vi "RunFullWormContinuousGWN.vi"() -> ()   [LabVIEW 2019]
uses:
  Parameters.ctl
  FullWormGWNClass/FullWormGWNInputCluster.ctl
  FullWormGWN.lvclass
  C:/Users/mochil/Dropbox/LeiferShaevitz/Github/ProjectAPI/LabviewVIs/StimulusObject.lvclass
panel:
  in  "FullWormGWNInputCluster":T1={"offset (red uW/mm^2m, blue is negative)"=0.0, "correlation time (s)"=0.5, "standard deviation (red uW/mm^2)"=70.0, "Max blue stimulus (uW/mm^2)"=130.0, "Max red stimulus (uW/mm^2)"=45.0, "dot radius (mm)"=0.3} {"Max red stimulus (uW/mm^2)" format="%#_13g"; "Max blue stimulus (uW/mm^2)" format="%#_13g"; "standard deviation (red uW/mm^2)" format="%#_13g"; "correlation time (s)" format="%#_13g"; "offset (red uW/mm^2m, blue is negative)" format="%#_13g"}
  out "error IO":errorcluster
  in  "Start":bool
  in  "Wait Before Recording (s)":u32
  in  "SSH password":string
  in  "SSH user name":string
  in  "Last Experiment of the Day":bool
  in  "Tags":string
  out "Parameters":T2 {"FW_WormLengthSD" format="%#.6e"}
  # "Faux Worm Drawing"
  # "Tracking"
  # "Temporal Calibration"
  # "Stimulus Generation"
  # "Median Filtering"
  # "Experimental Settings"
  # "Camera and Projector Settings"
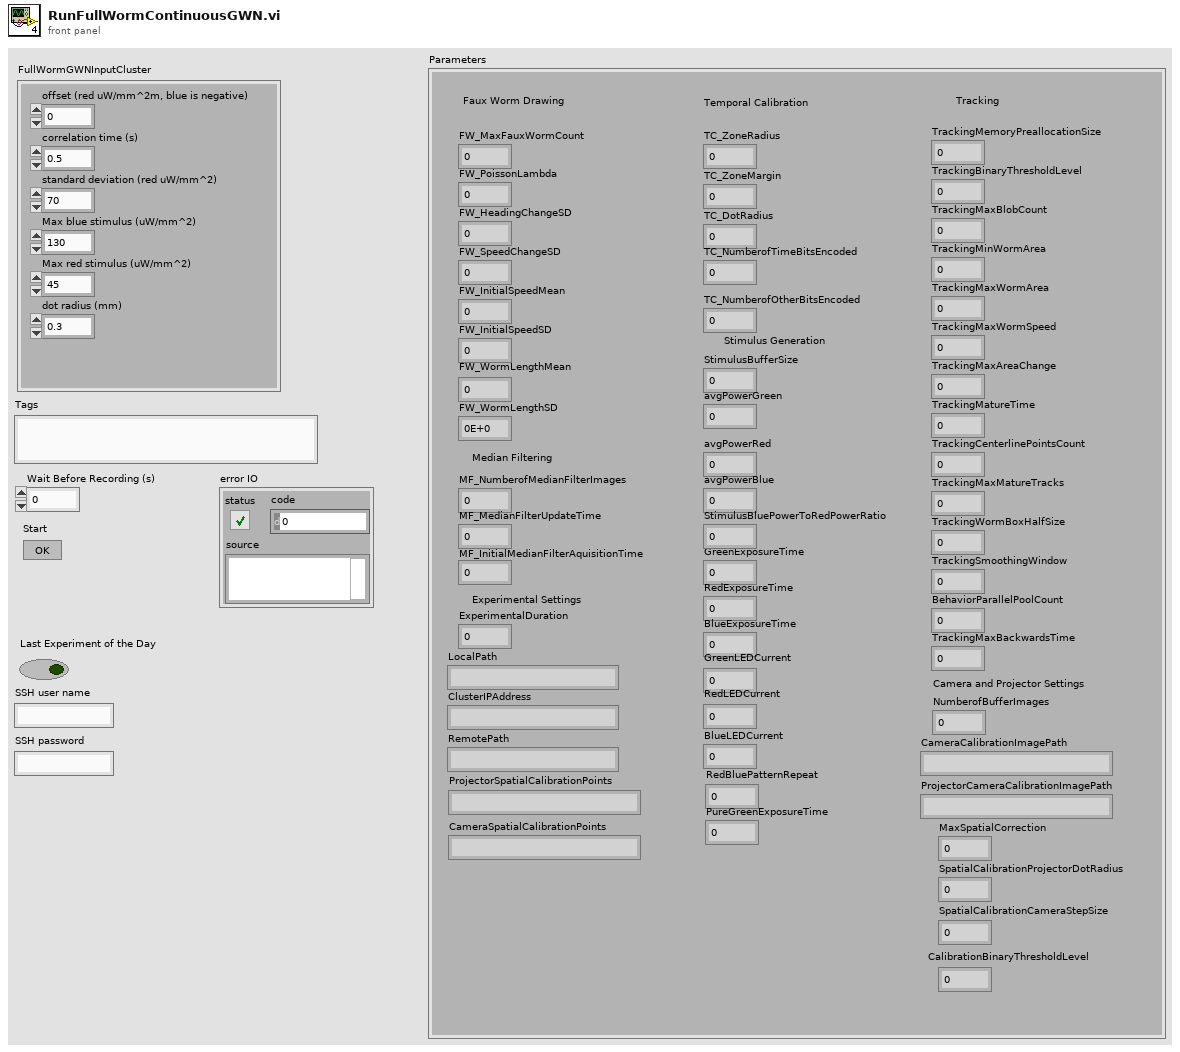
[diagram p1: front panel]
types:
  T1 = typedef "FullWormGWN.lvclass/FullWormGWNInputCluster.ctl" = cluster{"offset (red uW/mm^2m, blue is negative)":sgl, "correlation time (s)":sgl, "standard deviation (red uW/mm^2)":sgl, "Max blue stimulus (uW/mm^2)":sgl, "Max red stimulus (uW/mm^2)":sgl, "dot radius (mm)":sgl}
  T2 = typedef "Parameters.ctl" = cluster{"FW_MaxFauxWormCount":i32, "FW_PoissonLambda":dbl, "FW_HeadingChangeSD":dbl, "FW_SpeedChangeSD":dbl, "FW_InitialSpeedMean":dbl, "FW_InitialSpeedSD":dbl, "FW_WormLengthMean":dbl, "FW_WormLengthSD":dbl, "MF_NumberofMedianFilterImages":i32, "MF_MedianFilterUpdateTime":i32, "MF_InitialMedianFilterAquisitionTime":dbl, "ExperimentalDuration":i32, "TC_ZoneRadius":i32, "TC_ZoneMargin":i32, "TC_DotRadius":dbl, "TC_NumberofTimeBitsEncoded":i32, "TC_NumberofOtherBitsEncoded":i32, "NumberofBufferImages":sgl, "CameraCalibrationImagePath":string, "ProjectorCameraCalibrationImagePath":string, "StimulusBufferSize":i32, "TrackingMemoryPreallocationSize":i32, "TrackingBinaryThresholdLevel":sgl, "TrackingMaxBlobCount":i32, "TrackingMinWormArea":dbl, "TrackingMaxWormArea":dbl, "TrackingMaxWormSpeed":dbl, "TrackingMaxAreaChange":dbl, "TrackingMatureTime":i32, "TrackingCenterlinePointsCount":i32, "TrackingMaxMatureTracks":i32, "TrackingWormBoxHalfSize":i32, "TrackingSmoothingWindow":i32, "BehaviorParallelPoolCount":i32, "LocalPath":string, "GreenExposureTime":i32, "RedExposureTime":i32, "BlueExposureTime":i32, "ClusterIPAddress":string, "RemotePath":string, "GreenLEDCurrent":u8, "RedLEDCurrent":u8, "BlueLEDCurrent":u8, "avgPowerGreen":sgl, "avgPowerRed":sgl, "avgPowerBlue":sgl, "StimulusBluePowerToRedPowerRatio":sgl, "TrackingMaxBackwardsTime":i32, "MaxSpatialCorrection":dbl, "ProjectorSpatialCalibrationPoints":string, "SpatialCalibrationProjectorDotRadius":i32, "SpatialCalibrationCameraStepSize":dbl, "CameraSpatialCalibrationPoints":string, "CalibrationBinaryThresholdLevel":dbl, "RedBluePatternRepeat":i32, "PureGreenExposureTime":i32}
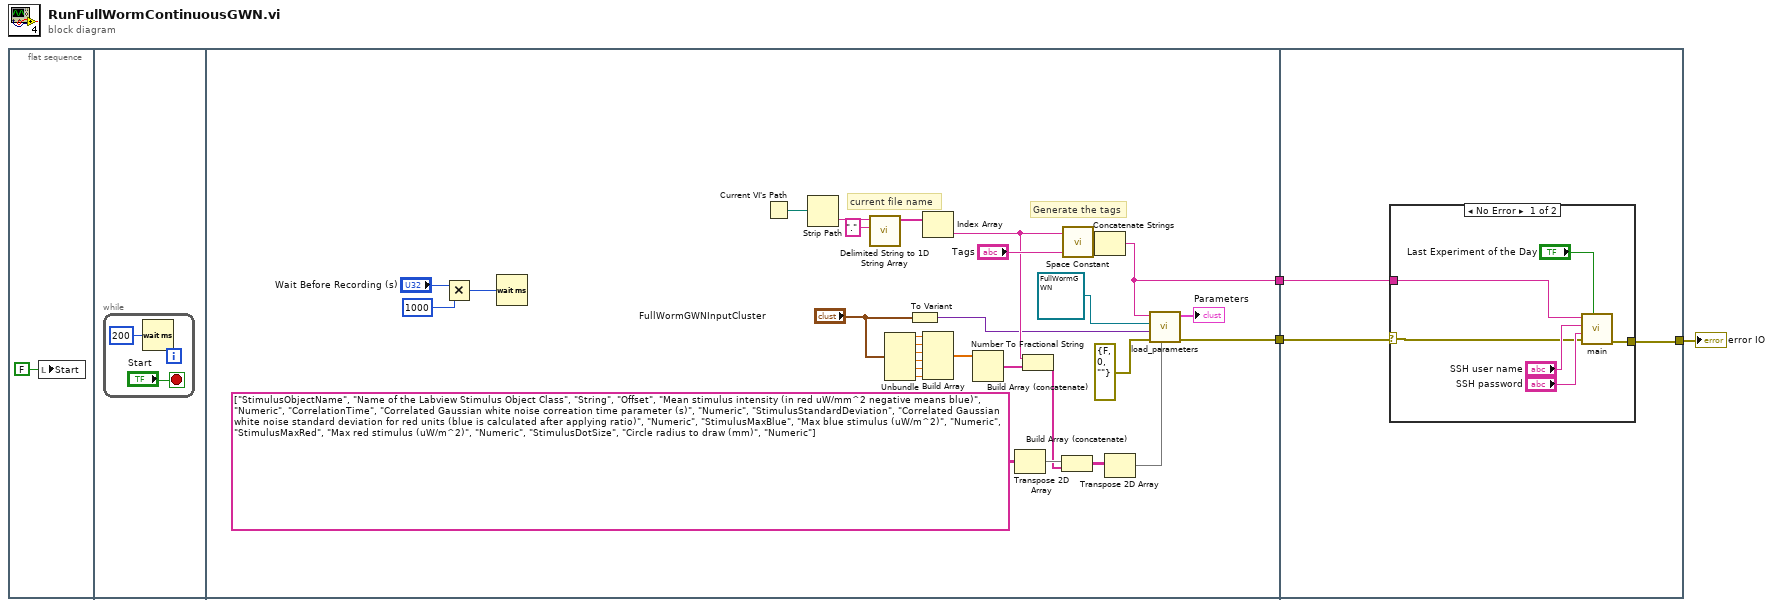
[diagram p0: block diagram]
diagram:
  n1 = flat-sequence {
    tunnel: [w36] -> w3
    tunnel: [w25] -> w2
    tunnel: w2 -> [w38]
    tunnel: w3 -> [w39]
    tunnel: [w37] -> w1
    frame #0 {
      n2 = local write "Start"(FALSE ("Start")) -> ()
    }
    frame #1 {
      n3 = while {
        stop <- "Start" stop-if-true
        n4 = Wait (ms)(milliseconds to wait=u32 200) -> ()  [unwired: 1 out]
      }
    }
    frame #2 {
      # "current file name"
      # "Generate the tags"
      n5 = Multiply(x="Wait Before Recording (s)", y=u32 1000) -> (x*y=w22:u32)
      n6 = Wait (ms)(milliseconds to wait=w22) -> ()  [unwired: 1 out]
      n7 = Current VI's Path() -> (path=w20:path)
      n8 = Strip Path(path=w20) -> (name=w19:string)  [unwired: 1 out]
      n9 = call <vilib>:"Delimited String to 1D String Array.vi"("delimiter"=".", "delimited string"=w19) -> ("string array"=w17:string[])  [unwired: 9 in]
      n10 = Unbundle("FullWormGWNInputCluster") -> ("offset (red uW/mm^2m, blue is negative)"=w15:sgl, "correlation time (s)"=w14:sgl, "standard deviation (red uW/mm^2)"=w13:sgl, "Max blue stimulus (uW/mm^2)"=w12:sgl, "Max red stimulus (uW/mm^2)"=w11:sgl, "dot radius (mm)"=w10:sgl)
      n11 = To Variant(anything="FullWormGWNInputCluster") -> (Variant=w8:variant)
      n12 = Index Array(array=w17) -> (element=w16:string)  [unwired: 1 in]
      n13 = Build Array(w15, w14, w13, w12, w11, w10) -> (w34:sgl[])
      n14 = Number To Fractional String(number=w34) -> (F-format string=w33:string[])  [unwired: 3 in]
      n15 = Transpose 2D Array(2D array=string[][] [["StimulusObjectName", "Name of the Labview Stimulus Object Class", "String"], ["Offset", "Mean stimulus intensity (in red uW/mm^2 negative means blue)", "Numeric"], ["CorrelationTime", "Correlated Gaussian white noise correation time parameter (s)", "Numeric"], ["StimulusStandardDeviation", "Correlated Gaussian white noise standard deviation for red units (blue is calculated after applying ratio)", "Numeric"], ["StimulusMaxBlue", "Max blue stimulus (uW/m^2)", "Numeric"], ["StimulusMaxRed", "Max red stimulus (uW/m^2)", "Numeric"], ["StimulusDotSize", "Circle radius to draw (mm)", "Numeric"]]) -> (transposed array=w31:string[][])
      n16 = Build Array (concatenate)(w16, w33) -> (w30:string[])
      n17 = Build Array (concatenate)(w31, w30) -> (w29:string[][])
      n18 = call <vilib>:"Space Constant.vi"() -> ("String"=w27:string)
      n19 = Concatenate Strings(w16, w27, "Tags") -> (w25:string)
      n20 = Transpose 2D Array(2D array=w29) -> (transposed array=w26:string[][])
      n21 = call "load_parameters.vi"("additional loaded parameters to write"=w26, "error in (no error)"=errorcluster {"status"=FALSE, "code"=0, "source"=""}, "StimulusObject Parameters"=w8, "StimulusObjectClassInput"=refnum<class "FullWormGWN.lvclass"> refnum ("FullWormGWN.lvclass"), "Tags"=w25) -> ("error out"=w36:errorcluster, "Parameters"=→"Parameters":T2)  [unwired: 4 in, 1 out]
    }
    frame #3 {
      n22 = case shown="No Error" w39 {
        selector: w39 -> [w42 w46]
        tunnel: [w41 w46] -> w37
        tunnel: w38 -> [w40 _]
        frame No Error {
          n23 = call "main.vi"("Last Experiment of the Day"="Last Experiment of the Day", "error in"=w42, "SSH password"="SSH password", "SSH user name"="SSH user name", "Tags"=w40) -> ("error out"=w41:errorcluster)  [unwired: 6 in]
        }
        frame Error {
        }
      }
    }
  }
  "error IO" <- w1
